vi "FindSerializableDataTypedef.vi"(8 "error in (no error)":errorcluster, 9 "Private data cluster refnum":refnum<vi>, 10 "LVClass refnum":refnum<vi>, 11 "SaveTo Path":path) -> (0 "error out":errorcluster, 1 "ctl is in class library?":bool, 2 "ctl File exists?":bool, 3 "SaveTo Path":path, 4 "ctl is in private data?":bool)   [LabVIEW 2019, in "BlueSerializationScripts.lvlib"]
uses:
  BlueSerializationScripts.lvlib
  BlueUtilityScripts/GetDescendantOptions.ctl
  8bd6079c-254c-4d1c-8b84-07c531051010.vi
  8bd6079c-254c-4d1c-8b84-07c531051010.vi/77e2fa99-364a-440c-b093-303216b3ba27.vi
  <userlib>/_OpenG.lib/file/file.llb/File Exists - Scalar__ogtk.vi
  BlueSerialProviderGlobal.vi
  BlueUtilityScripts/BlueUtilityScripts.lvlib
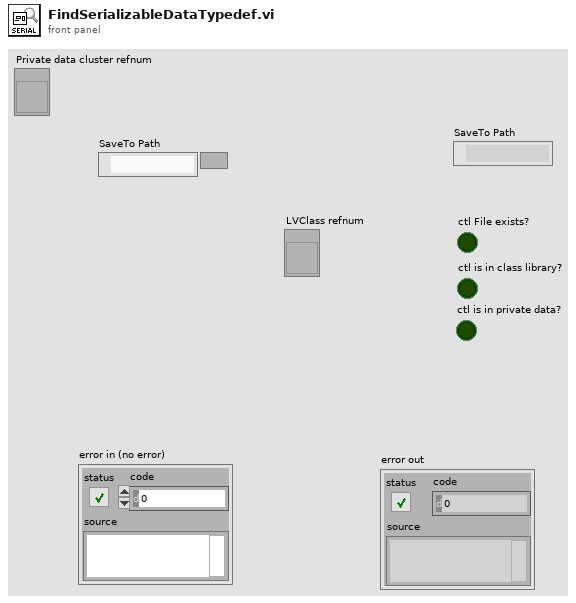
[diagram p1: front panel]
types:
  T1 = typedef "BlueUtilityScripts.lvlib/GetDescendantOptions.ctl" = cluster{"Type":string, "ExcludeDependencies":bool, "ExcludeBuilds":bool, "ExcludeTargets":bool}
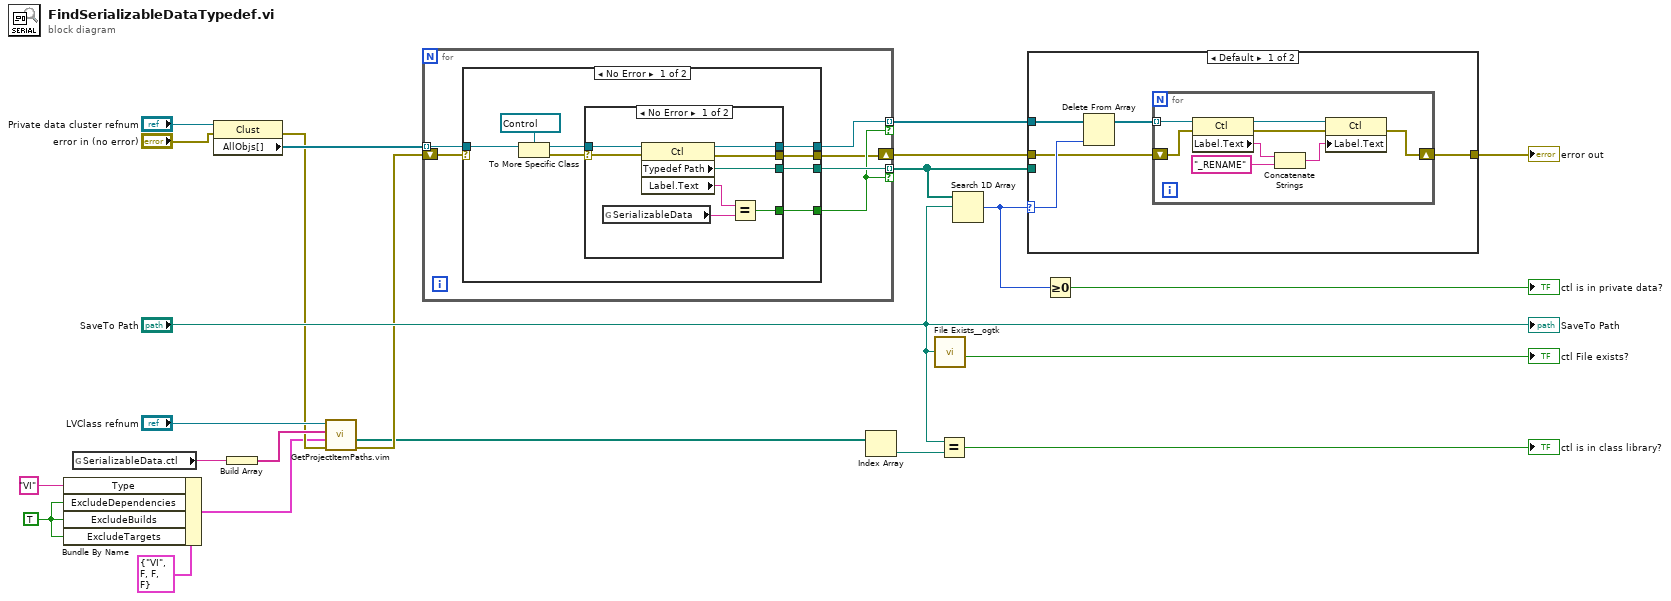
[diagram p0: block diagram]
diagram:
  w2 = TRUE ("ExcludeBuilds")
  n1 = Bundle By Name(cluster=T1 {"Type"="VI", "ExcludeDependencies"=FALSE, "ExcludeBuilds"=FALSE, "ExcludeTargets"=FALSE} ("Search Options"), "Type"="VI", "ExcludeDependencies"=w2, "ExcludeBuilds"=w2, "ExcludeTargets"=w2) -> (w1:T1)
  n2 = global read "BlueSerialProviderGlobal.vi" "SerializableData.ctl"() -> (w9:string)
  n3 = property class="Clust"(reference="Private data cluster refnum", error in="error in (no error)") -> (error out=w11:errorcluster, "AllObjs[]"=w21:refnum<vi>[])  [unwired: 1 out]
  n4 = Build Array(w9) -> (w18:string[])
  n5 = call "GetProjectItemPaths.vim"("error in (no error)"=w11, "Search Options"=w1, "Item Name"=w18, "ProjectItem"="LVClass refnum") -> ("error out"=w7:errorcluster, "Paths"=w5:path[])  [unwired: 4 in, 2 out]
  n6 = for {
    tunnel: w21 -> [w28] mode=indexing
    tunnel: [w29] -> w22 mode=indexing if=w27
    tunnel: [w26] -> w8 mode=indexing if=w27
    shift-right: [w25] -> w6
    shift-left: w7 -> [w24]
    n7 = case shown="No Error" w24 {
      selector: w24 -> [_ w46]
      tunnel: [w36 _] -> w29
      tunnel: w28 -> [w33 _]
      tunnel: [w32 _] -> w27
      tunnel: [w31 _] -> w26
      tunnel: [w30 w46] -> w25
      frame No Error {
        n8 = To More Specific Class(target class=refnum<vi> refnum ("element"), reference=w33) -> (specific class reference=w34:refnum<vi>, error out=w35:errorcluster)  [unwired: 1 in]
        n9 = case shown="No Error" w35 {
          selector: w35 -> [w42 _]
          tunnel: [w45 _] -> w36
          tunnel: w34 -> [w41 _]
          tunnel: [w40 _] -> w32
          tunnel: [w39 _] -> w30
          tunnel: [w38 _] -> w31
          frame No Error {
            n10 = global read "BlueSerialProviderGlobal.vi" "SerializableData"() -> (w44:string)
            n11 = property class="Ctl"(reference=w41, error in=w42) -> (reference out=w38:refnum<vi>, error out=w39:errorcluster, "Typedef Path"=w45:path, "Label.Text"=w43:string)
            n12 = Equal?(x=w43, y=w44) -> (x = y?=w40:bool)
          }
          frame Error {
          }
        }
      }
      frame Error {
      }
    }
  }
  n13 = Index Array(array=w5) -> (element=w17:path)  [unwired: 1 in]
  n14 = call-poly <userlib>:"File Exists__ogtk.vi"("file path"="SaveTo Path") -> ("exists"=→"ctl File exists?":bool)  [unwired: 6 in, 1 out]
  n15 = Equal?(x="SaveTo Path", y=w17) -> (x = y?=→"ctl is in class library?":bool)
  n16 = Search 1D Array(1D array=w22, element="SaveTo Path") -> (index of element=w14:i32)  [unwired: 1 in]
  n17 = case shown="Default" w14 {
    selector: w14 -> [w50 _]
    tunnel: w22 -> [_ _]
    tunnel: w8 -> [w51 _]
    tunnel: w6 -> [w48 w60]
    tunnel: [w47 w60] -> w10
    frame Default {
      n18 = Delete From Array(array=w51, index=w50) -> (array with subset deleted=w49:refnum<vi>[])  [unwired: 1 in, 1 out]
      n19 = for {
        tunnel: w49 -> [w59] mode=indexing
        shift-right: [w52] -> w47
        shift-left: w48 -> [w55]
        n20 = property class="Ctl"(reference=w59, error in=w55) -> (reference out=w58:refnum<vi>, error out=w54:errorcluster, "Label.Text"=w57:string)
        n21 = Concatenate Strings(w57, "_RENAME" ("string")) -> (w53:string)
        n22 = property class="Ctl"(reference=w58, error in=w54, "Label.Text"=w53) -> (error out=w52:errorcluster)  [unwired: 1 out]
      }
    }
    frame -1 {
    }
  }
  "error out" <- w10
  n23 = Greater Or Equal To 0?(x=w14) -> (x >= 0?=→"ctl is in private data?":bool)
  "SaveTo Path" <- "SaveTo Path"
